vi "basement tank animations.vi"() -> ()   [LabVIEW 2018]
panel:
  in  "Enable T Control":bool
  in  "Enable Main Pump":bool
  out "Boolean 6":bool
  out "Temperature":dbl
  out "Boolean 5":bool
  out "Boolean 4":bool
  out "Boolean 3":bool
  out "Circulator":bool
  out "Boolean":bool
  out "Tank":dbl(slide) scale=0.0..250.0
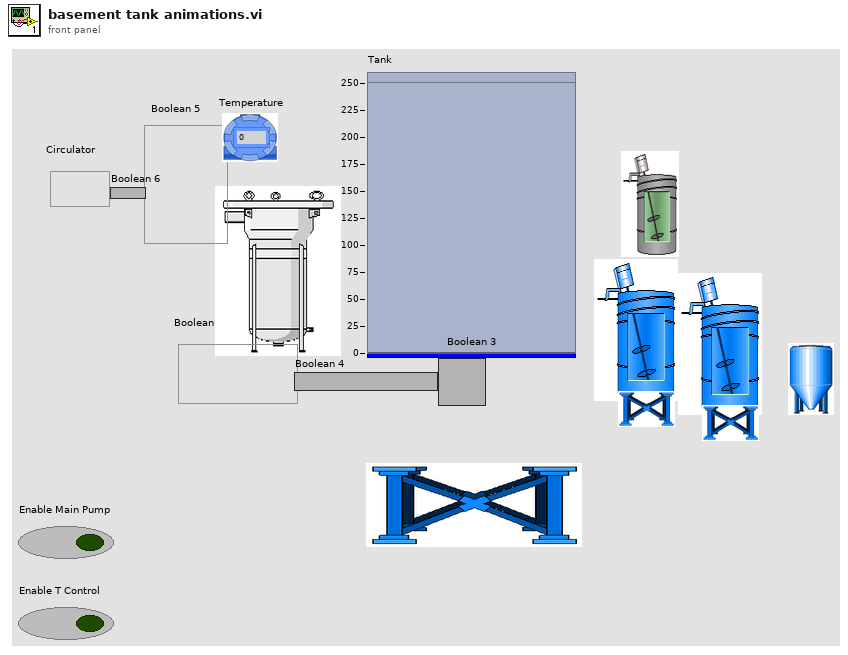
[diagram p1: front panel]
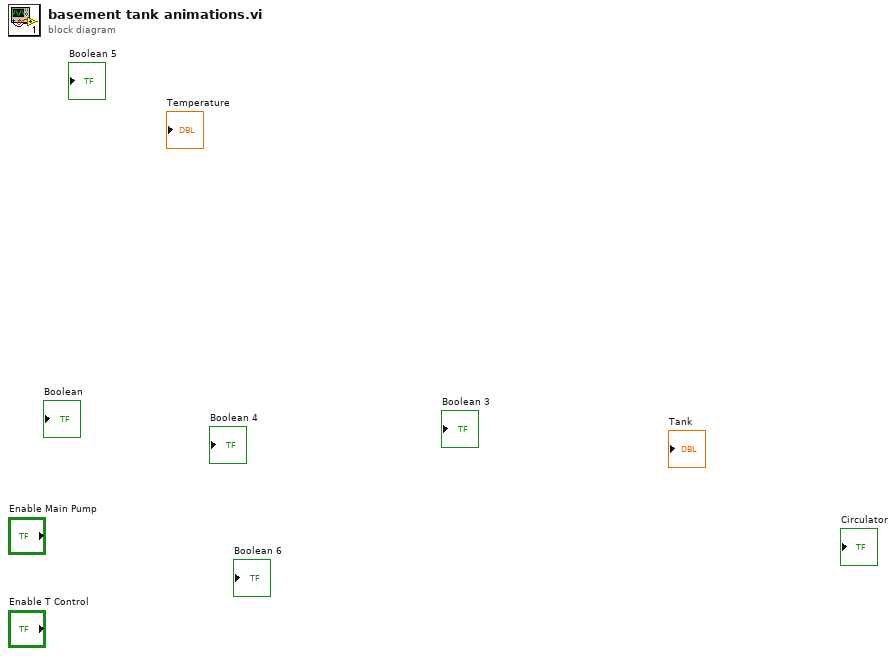
[diagram p0: block diagram]
diagram:
